vi "add channel to configuration.vi"(8 "error in":errorcluster, 10 "Modbus Module Channel.lvclass":refnum<class "Modbus Module Channel.lvclass">, 11 "Modbus Slave configuration in":refnum<class "Modbus Slave configuration.lvclass">) -> (0 "error out":errorcluster, 3 "Modbus Slave configuration out":refnum<class "Modbus Slave configuration.lvclass">)   [LabVIEW 2013, in "Modbus Slave configuration.lvclass"]
doc: "Platypus Framework 1.0.1.65\nNI Systems Engineering - National Instruments"
uses:
  Modbus Slave configuration.lvclass
  module channel/Modbus Module Channel.lvclass
  <vilib>/NI/Tag Bus/tag/tag descriptor.lvclass/tag descriptor.ctl
  Modbus Slave configuration.lvclass/Modbus Slave configuration.ctl
  <vilib>/NI/Tag Bus/tag/tag descriptor.lvclass
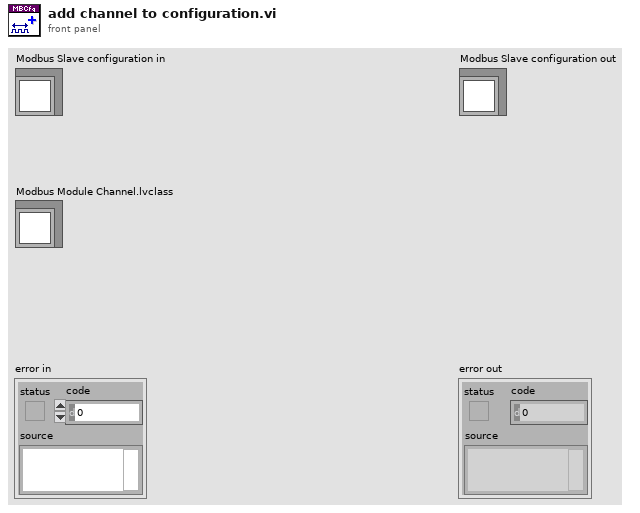
[diagram p1: front panel]
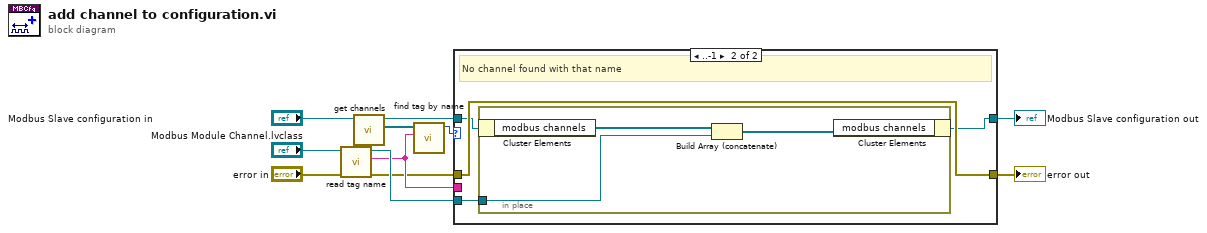
[diagram p0: block diagram]
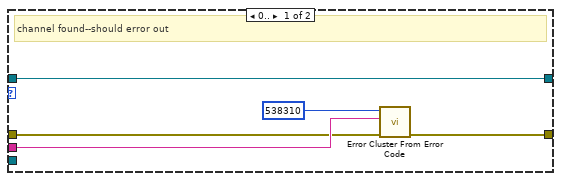
[diagram p2: hidden frame]
diagram:
  n1 = call <vilib>:"read tag name.vi"("error in"="error in", "system tag in"="Modbus Module Channel.lvclass") -> ("error out"=w2:errorcluster, "name"=w3:string, "system tag out"=w10:refnum<class "Modbus Module Channel.lvclass">)  [unwired: 7 in]
  n2 = call-dynamic "get channels.vi"("Modbus Slave configuration in"="Modbus Slave configuration in") -> ("channels"=w5:refnum<class "TBM channel.lvclass">[], "Modbus Slave configuration out"=w11:refnum<class "Modbus Slave configuration.lvclass">)  [unwired: 9 in]
  n3 = call <vilib>:"find tag by name.vi"("name"=w3, "tags in"=w5) -> ("index"=w4:i32)  [unwired: 9 in]
  n4 = case shown="..-1" w4 {
    tunnel: [w16 w19] -> w8
    tunnel: w3 -> [w14 _]
    tunnel: w2 -> [w13 w19]
    tunnel: w11 -> [w12 w18]
    tunnel: w10 -> [_ w20]
    tunnel: [w12 w17] -> w7
    frame 0.. {
      # "channel found--should error out"
      n5 = call <vilib>:"Error Cluster From Error Code.vi"("error in (no error)"=w13, "error message (\"\")"=w14, "error code (0)"=538310) -> ("error out"=w16:errorcluster)  [unwired: 6 in]
    }
    frame ..-1 {
      # "No channel found with that name"
      n6 = in-place {
        in-place-border: w20 -> [w23]
        n7 = in-place-cluster #1(w18) -> ("modbus channels"=w21:refnum<class "Modbus Module Channel.lvclass">[])
        n8 = Build Array (concatenate)(w21, w23) -> (w22:refnum<class "Modbus Module Channel.lvclass">[])
        n9 = in-place-cluster #1("modbus channels"=w22) -> (w17:refnum<class "Modbus Slave configuration.lvclass">)
      }
    }
  }
  "error out" <- w8
  "Modbus Slave configuration out" <- w7
